vi "Create table if not exists.vi"(8 "error in (no error)":errorcluster, 11 "IConfigDBQueries in":refnum<class "sqlite-queries.lvclass">) -> (0 "error out":errorcluster, 2 "Query out":string)   [LabVIEW 2020, in "sqlite-queries.lvlib" / "sqlite-queries.lvclass"]
uses:
  sqlite-queries.lvclass
  sqlite-queries.lvclass/sqlite-queries.ctl
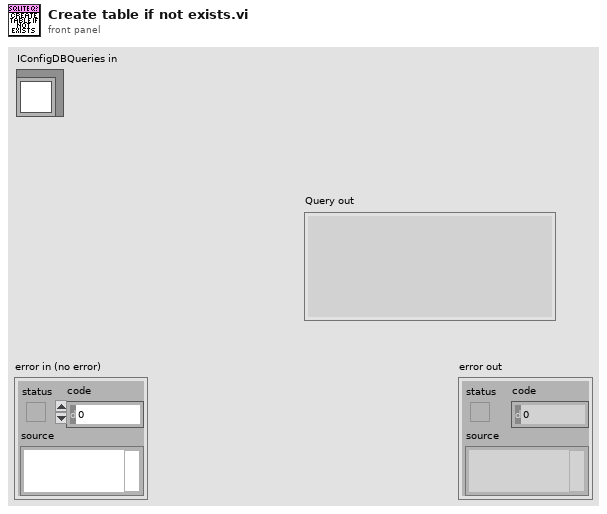
[diagram p1: front panel]
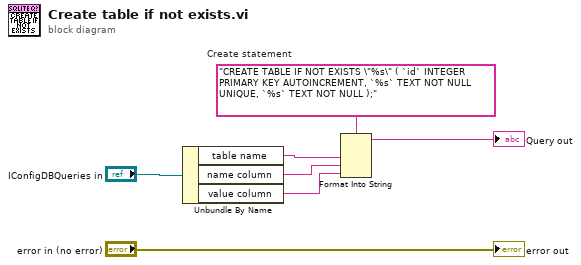
[diagram p0: block diagram]
diagram:
  w5 = "CREATE TABLE IF NOT EXISTS \"%s\" ( `id` INTEGER PRIMARY KEY AUTOINCREMENT, `%s` TEXT NOT NULL UNIQUE, `%s` TEXT NOT NULL );"  # Create statement
  n1 = Unbundle By Name("IConfigDBQueries in") -> ("table name"=w4:string, "name column"=w3:string, "value column"=w2:string)
  n2 = Format Into String(format string=w5, w4, w3, w2) -> (resulting string=→"Query out":string)  [unwired: 2 in, 1 out]
  "error out" <- "error in (no error)"
